vi "Picture_Clock_Main.vi"(9 "Picture-Time / [ms]":dbl, 10 "Source":tag="/Dev2/PFI0" caption="Picture Start Clock in", 11 "Counter(s)":tag="Dev1/ctr1" caption="Picture Clock Main out") -> (0 "error out":errorcluster, 2 "Number of Pulses per Picture / [x1 us]":i32, 3 "task out":refnum<k21>)   [LabVIEW 2009]
uses:
  <vilib>/DAQmx/configure/trigger.llb/DAQmx Start Trigger (Digital Edge).vi
  <vilib>/DAQmx/configure/timing.llb/DAQmx Timing (Implicit).vi
  <vilib>/DAQmx/create/channels.llb/DAQmx Create Channel (CO-Pulse Generation-Frequency).vi
  Program Files/National Instruments/LabVIEW 2009/resource/objmgr/daqmx.rc
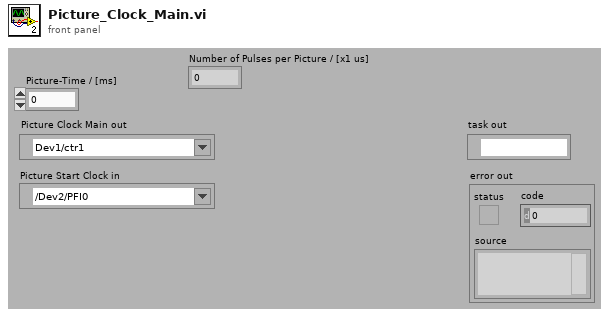
[diagram p1: front panel]
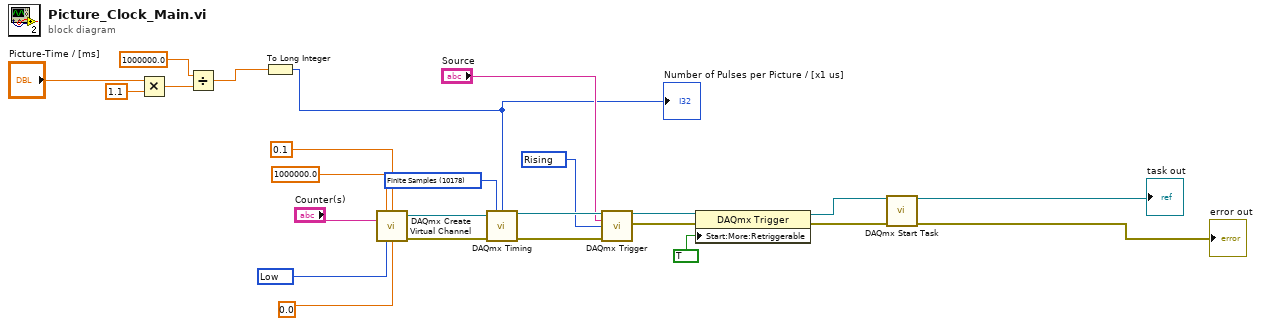
[diagram p0: block diagram]
diagram:
  w15 = 10280 items=["Rising"=10280, "Falling"=10171] ("Trigger Edge")
  w21 = 10214 items=["High"=10192, "Low"=10214] ("Idle State")
  w23 = 10178 items=["Finite Samples"=10178, "Continuous Samples"=10123] ("sample mode")
  n1 = Multiply(x="Picture-Time / [ms]", y=1.1) -> (x*y=w4:dbl)
  n2 = Divide(x=1000000.0 ("y"), y=w4) -> (x/y=w3:dbl)
  n3 = To Long Integer(number=w3) -> (32bit integer=w1:i32)
  "Number of Pulses per Picture / [x1 us]" <- w1
  n4 = call-poly <vilib>:"DAQmx Create Virtual Channel.vi"("frequency"=1000000.0 ("Frequency"), "duty cycle"=0.1 ("Duty Cycle"), "counter"="Counter(s)", "idle state"=w21, "initial delay"=0.0 ("Initial delay")) -> ("task out"=w24:refnum<k21>, "error out"=w25:errorcluster)  [unwired: 4 in, 5 out]
  n5 = call-poly <vilib>:"DAQmx Timing.vi"("task/channels in"=w24, "sample mode"=w23, "samples per channel"=w1, "error in"=w25) -> ("task out"=w17:refnum<k21>, "error out"=w16:errorcluster)  [unwired: 2 in, 8 out]
  n6 = call-poly <vilib>:"DAQmx Trigger.vi"("task/channels in"=w17, "source"="Source", "edge"=w15, "error in"=w16) -> ("task out"=w13:refnum<k21>, "error out"=w12:errorcluster)  [unwired: 10 out]
  n7 = property class="DAQmx Trigger"(reference=w13, error in=w12, "Start:More:Retriggerable"=TRUE) -> (reference out=w11:refnum<k21>, error out=w10:errorcluster)
  n8 = call <vilib>:"DAQmx Start Task.vi"("task/channels in"=w11, "error in"=w10) -> ("task out"=→"task out":refnum<k21>, "error out"=→"error out":errorcluster)  [unwired: 12 out]
